vi "Mod_OFDM_Write_Configuration_To_File.vi"(0 "Configuration in":variant, 11 "error in":errorcluster) -> (4 "Configuration out":variant, 15 "error out":errorcluster)   [LabVIEW 2010]
doc: "Stores the current configuration in an .ofm file which can be read back by the \"Mod_OFDM_Read_Configuration_From_File\" VI."
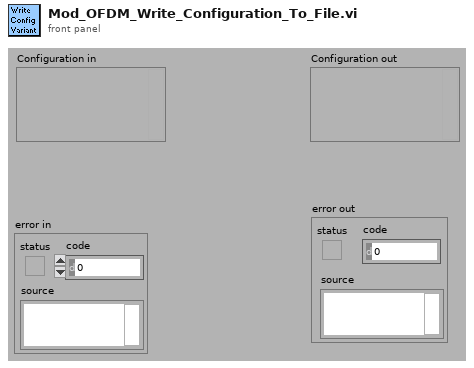
[diagram p1: front panel]
types:
  T1 = enum16{"open", "open or create", "create or replace", "create", "open (read only)"}
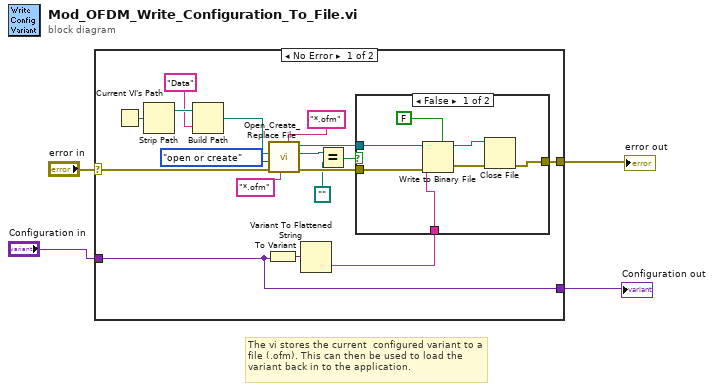
[diagram p0: block diagram]
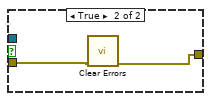
[diagram p2: hidden frame]
diagram:
  # "The vi stores the current  configured variant to a file (.ofm). This can then be used to load the variant back in to the application."
  n1 = case shown="No Error" "error in" {
    selector: "error in" -> [w12 w31]
    tunnel: [w14 w31] -> w4
    tunnel: "Configuration in" -> [w13 _]
    tunnel: [w13 _] -> w2
    frame No Error {
      n2 = Current VI's Path() -> (path=w11:path)
      n3 = Strip Path(path=w11) -> (stripped path=w10:path)  [unwired: 1 out]
      n4 = Build Path(base path=w10, name or relative path="Data") -> (appended path=w8:path)
      n5 = To Variant(anything=w13) -> (Variant=w21:variant)
      n6 = call <vilib>:"Open_Create_Replace File.vi"("pattern"="*.ofm", "default name"="*.ofm", "error in (no error)"=w12, "function (open:0)"=T1."open or create", "start path  (Not A Path)"=w8) -> ("error out"=w16:errorcluster, "new file path"=w6:path, "refnum"=w17:refnum<file>)  [unwired: 3 in, 1 out]
      n7 = Variant To Flattened String(Variant=w21) -> (data string=w15:string)  [unwired: 1 out]
      n8 = Equal?(x=w6, y=path "") -> (x = y?=w7:bool)
      n9 = case shown="False" w7 {
        tunnel: w17 -> [w28 _]
        tunnel: w16 -> [w27 w30]
        tunnel: w15 -> [w26 _]
        tunnel: [w24 w29] -> w14
        frame False {
          n10 = Write to Binary File(file (use dialog)=w28, data=w26, error in=w27, 5:FALSE ("prepend array or string size? (T)")) -> (refnum out=w25:refnum<file>, error out=w23:errorcluster)  [unwired: 2 in, 1 out]
          n11 = Close File(refnum=w25, error in=w23) -> (error out=w24:errorcluster)  [unwired: 1 out]
        }
        frame True {
          n12 = call <vilib>:"Clear Errors.vi"("error in (no error)"=w30) -> ("error out"=w29:errorcluster)  [unwired: 6 in]
        }
      }
    }
    frame Error {
    }
  }
  "Configuration out" <- w2
  "error out" <- w4
